vi "tri.vi"(9 "t2":dbl, 10 "dt(s)":dbl, 11 "i":i32) -> (0 "t2?":bool, 1 "complet?":bool, 2 "Waveform Chart":dbl(graph), 4 "t3":dbl)   [LabVIEW 2019]
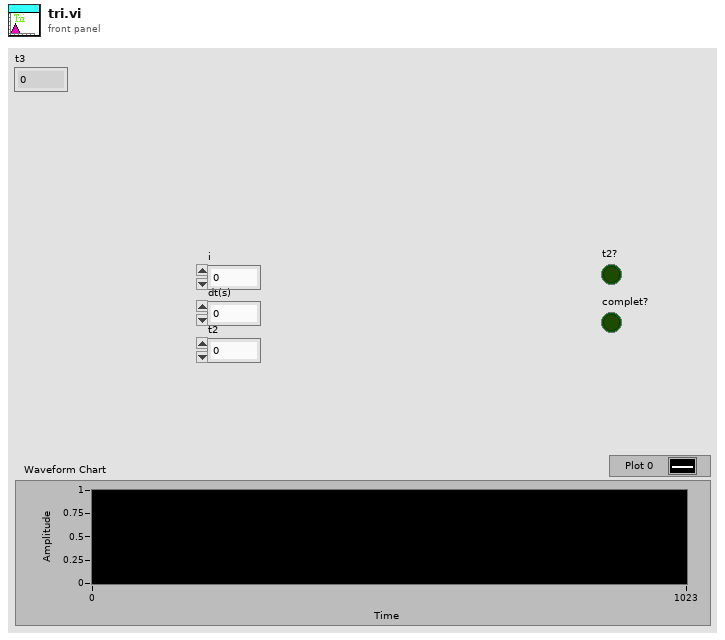
[diagram p1: front panel]
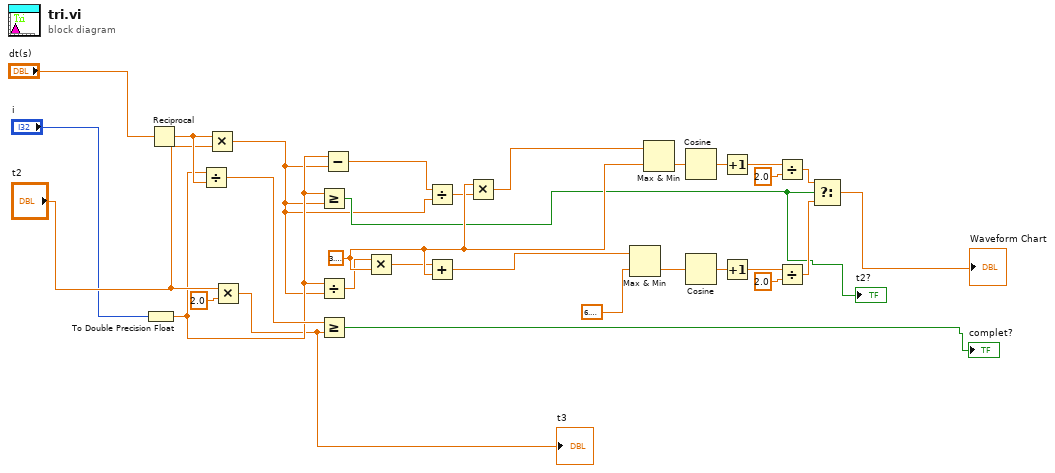
[diagram p0: block diagram]
diagram:
  w24 = 3.141592653589793
  n1 = To Double Precision Float(number="i") -> (double precision float=w4:dbl)
  n2 = Reciprocal(x="dt(s)") -> (1/x=w12:dbl)
  n3 = Divide(x=w4, y=w12) -> (x/y=w11:dbl)
  n4 = Multiply(x=w12, y="t2") -> (x*y=w3:dbl)
  n5 = Multiply(x="t2", y=2.0) -> (x*y=w1:dbl)
  "t3" <- w1
  n6 = Greater Or Equal?(x=w4, y=w3) -> (x >= y?=w5:bool)
  "t2?" <- w5
  n7 = Divide(x=w4, y=w3) -> (x/y=w13:dbl)
  n8 = Greater Or Equal?(x=w11, y=w1) -> (x >= y?=→"complet?":bool)
  n9 = Subtract(x=w4, y=w3) -> (x-y=w2:dbl)
  n10 = Multiply(x=w13, y=w24) -> (x*y=w15:dbl)
  n11 = Divide(x=w2, y=w3) -> (x/y=w22:dbl)
  n12 = Add(x=w15, y=w24) -> (x+y=w17:dbl)
  n13 = Multiply(x=w24, y=w22) -> (x*y=w23:dbl)
  n14 = Max & Min(x=w17, y=6.283185307179586) -> (min(x,y)=w18:dbl)  [unwired: 1 out]
  n15 = Max & Min(x=w23, y=w24) -> (min(x,y)=w25:dbl)  [unwired: 1 out]
  n16 = Cosine(x=w25) -> (cos(x)=w26:dbl)
  n17 = Cosine(x=w18) -> (cos(x)=w19:dbl)
  n18 = Increment(x=w26) -> (x+1=w27:dbl)
  n19 = Increment(x=w19) -> (x+1=w20:dbl)
  n20 = Divide(x=w27, y=2.0) -> (x/y=w30:dbl)
  n21 = Divide(x=w20, y=2.0) -> (x/y=w29:dbl)
  n22 = Select(t=w30, s=w5, f=w29) -> (s? t:f=→"Waveform Chart":dbl)
